vi "SetSettingsSingle.vi"(8 "error in (no error)":errorcluster, 11 "MagSpecCamera.lvclass":refnum<class "MagSpecCamera.lvclass">) -> (0 "error out":errorcluster, 3 "MagSpecCamera in":refnum<class "MagSpecCamera.lvclass">)   [LabVIEW 2020, in "MagSpecCamera.lvclass"]
uses:
  MagSpecCamera.lvclass
  OnOffTypeDef.ctl
  MagSpecCamera.lvclass/MagSpecCamera.ctl
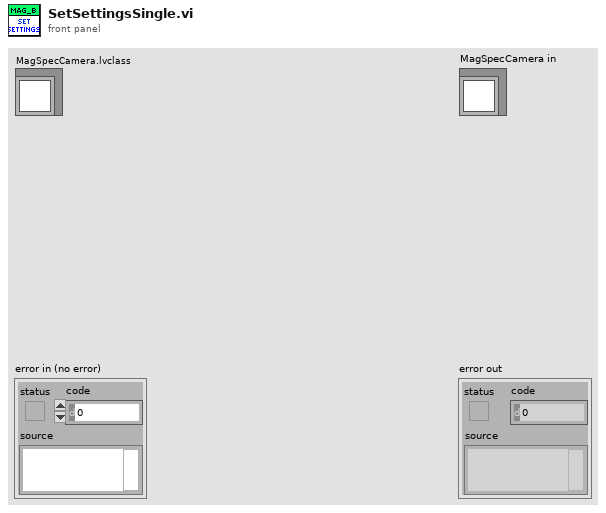
[diagram p1: front panel]
types:
  T1 = typedef "OnOffTypeDef.ctl" = enum16{"off", "on"}
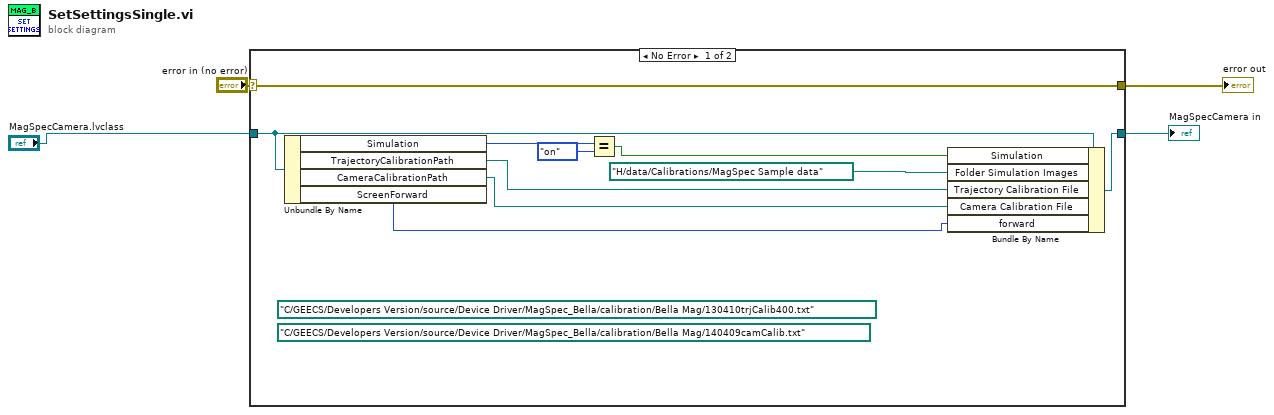
[diagram p0: block diagram]
diagram:
  n1 = case shown="No Error" "error in (no error)" {
    selector: "error in (no error)" -> [w14 w16]
    tunnel: [w14 w16] -> w3
    tunnel: [w12 w15] -> w2
    tunnel: "MagSpecCamera.lvclass" -> [w11 w15]
    frame No Error {
      (unwired) path "C:/GEECS/Developers Version/source/Device Driver/MagSpec_Bella/calibration/Bella Mag/140409camCalib.txt" ("Settings.Calibration Files.Camera Calibration File")
      (unwired) path "C:/GEECS/Developers Version/source/Device Driver/MagSpec_Bella/calibration/Bella Mag/130410trjCalib400.txt" ("Settings.Calibration Files.Trajectory Calibration File")
      n2 = Unbundle By Name(w11) -> ("Simulation"=w8:T1, "TrajectoryCalibrationPath"=w10:path, "CameraCalibrationPath"=w9:path, "ScreenForward"=w5:T1)
      n3 = Equal?(x=w8, y=OnOffTypeDef."on") -> (x = y?=w6:bool)
      n4 = Bundle By Name(cluster=w11, "Simulation"=w6, "Folder Simulation Images"=path "H:/data/Calibrations/MagSpec Sample data" ("Settings.Folder Simulation Images"), "Trajectory Calibration File"=w10, "Camera Calibration File"=w9, "forward"=w5) -> (w12:refnum<class "MagSpecCamera.lvclass">)
    }
    frame Error {
    }
  }
  "error out" <- w3
  "MagSpecCamera in" <- w2
